vi "SS Close.vi"(8 "error in (no error)":errorcluster, 11 "Subsystem Class in":refnum<class "Subsystem Class.lvclass">) -> (0 "error out":errorcluster, 3 "Subsystem Class out":refnum<class "Subsystem Class.lvclass">)   [LabVIEW 2021, in "Subsystem Class.lvclass"]
uses:
  Subsystem Class.lvclass
  SS typedef cluster Instrument Command Queue Data.ctl
  Subsystem Class.lvclass/Subsystem Class.ctl
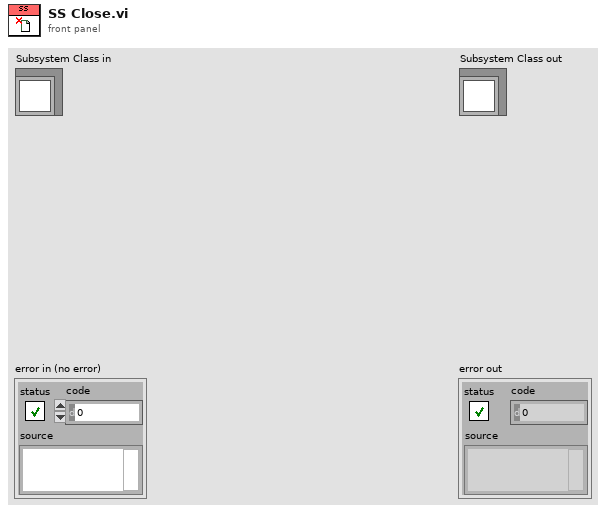
[diagram p1: front panel]
types:
  T1 = typedef "SS typedef cluster Instrument Command Queue Data.ctl" = cluster{"Cmd":string, "Parameters":variant}
  T2 = typedef "SS typedef Cmd Queue Reference.ctl" = refnum<queue>
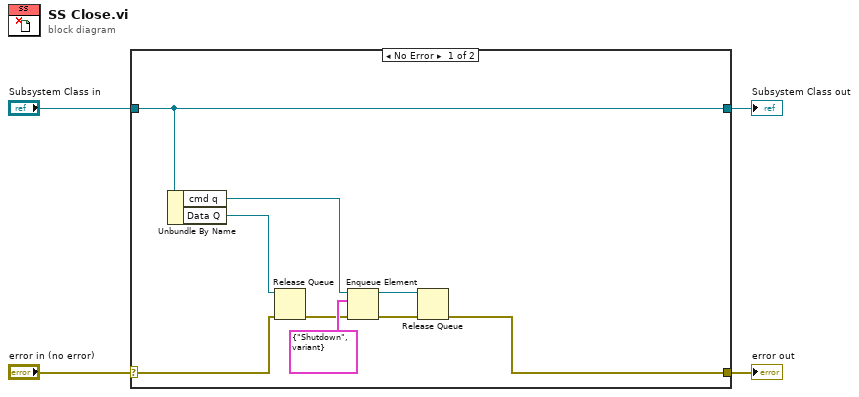
[diagram p0: block diagram]
diagram:
  n1 = case shown="No Error" "error in (no error)" {
    selector: "error in (no error)" -> [w12 w15]
    tunnel: [w5 w15] -> w3
    tunnel: [w13 w14] -> w1
    tunnel: "Subsystem Class in" -> [w13 w14]
    frame No Error {
      n2 = Unbundle By Name(w13) -> ("cmd q"=w9:T2, "Data Q"=w11:refnum<queue>)
      n3 = Release Queue(queue=w11, error in (no error)=w12) -> (error out=w8:errorcluster)  [unwired: 1 in, 2 out]
      n4 = Enqueue Element(queue=w9, element=T1 {"Cmd"="Shutdown", "Parameters"=variant}, error in (no error)=w8) -> (queue out=w6:T2, error out=w7:errorcluster)  [unwired: 1 in, 1 out]
      n5 = Release Queue(queue=w6, error in (no error)=w7) -> (error out=w5:errorcluster)  [unwired: 1 in, 2 out]
    }
    frame Error {
    }
  }
  "error out" <- w3
  "Subsystem Class out" <- w1
